vi "READ.vi"(8 "error in (no error)":errorcluster) -> (0 "error out":errorcluster, 3 "Monedas 2":T1(array[cluster]))   [LabVIEW 2020, in "Monedas.lvlib"]
uses:
  Monedas.lvlib
  <vilib>/Utility/xml.llb/Read From XML File(string).vi
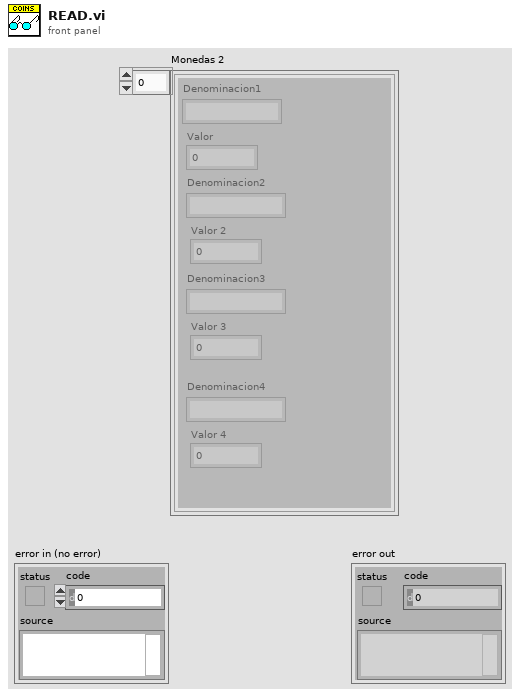
[diagram p1: front panel]
types:
  T1 = cluster{"Denominacion1":string, "Valor":dbl, "Denominacion2":string, "Valor 2":dbl, "Denominacion3":string, "Valor 3":dbl, "Denominacion4":string, "Valor 4":dbl}[]
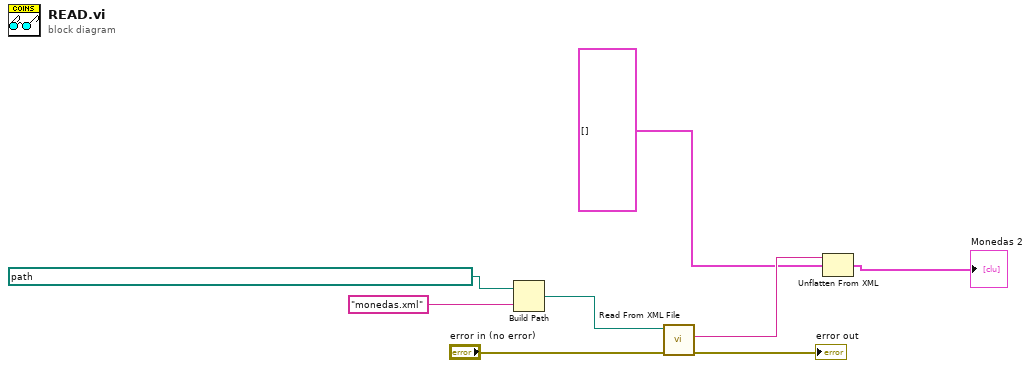
[diagram p0: block diagram]
diagram:
  n1 = Build Path(base path=path "C:/Users/Ymata/Desktop/séptimo/labview 7mo/Proyecto máuina/Proyecto-maquina", name or relative path="monedas.xml") -> (appended path=w4:path)
  n2 = call-poly <vilib>:"Read From XML File.vi"("error in (no error)"="error in (no error)", "XML File Path"=w4) -> ("error out"=→"error out":errorcluster, "XML Elements"=w8:string)  [unwired: 7 in, 1 out]
  n3 = Unflatten From XML(xml string=w8, type=T1 []) -> (value=→"Monedas 2":T1)  [unwired: 1 in, 1 out]
